vi "Auto 4.vi"(8 "Error In":errorcluster) -> (0 "Error Out":errorcluster)   [LabVIEW 2014]
uses:
  Robot Global Data.vi
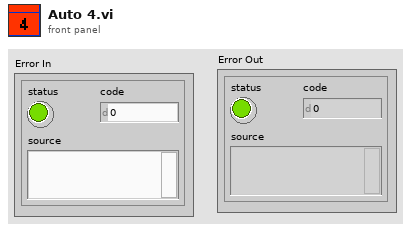
[diagram p1: front panel]
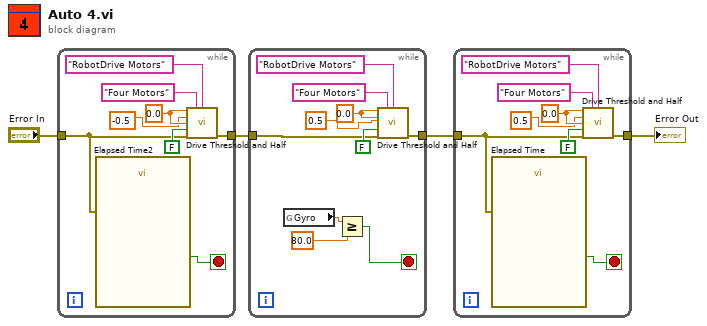
[diagram p0: block diagram]
diagram:
  n1 = while {
    tunnel: "Error In" -> [w5]
    tunnel: [w9] -> w3
    stop <- w6 stop-if-true
    w8 = 0.0 ("Arm Value")
    n2 = call "Elapsed Time2"("error in (no error)"=w5) -> ("Time has Elapsed"=w6:bool)  [unwired: 11 in, 7 out]
    n3 = call "Drive Threshold and Half.vi"("X In"=w8, "Drive refnum name"="Four Motors" ("refnum name"), "Send to DB Name"="RobotDrive Motors" ("Name"), "Y In"=-0.5 ("X In"), "R In"=w8, "Speed Toggle"=FALSE ("Grabber Open/Close"), "Error In"=w5) -> ("Error Out"=w9:errorcluster)  [unwired: 8 in]
  }
  n4 = while {
    tunnel: w3 -> [w19]
    tunnel: [w18] -> w4
    stop <- w13 stop-if-true
    w17 = 0.0 ("Arm Value")
    n5 = global read "Robot Global Data.vi" "Gyro"() -> (w15:dbl)
    n6 = Greater Or Equal?(x=w15, y=80.0) -> (x >= y?=w13:bool)
    n7 = call "Drive Threshold and Half.vi"("X In"=w17, "Drive refnum name"="Four Motors" ("refnum name"), "Send to DB Name"="RobotDrive Motors" ("Name"), "Y In"=w17, "R In"=0.5 ("X In"), "Speed Toggle"=FALSE ("Grabber Open/Close"), "Error In"=w19) -> ("Error Out"=w18:errorcluster)  [unwired: 8 in]
  }
  n8 = while {
    tunnel: w4 -> [w23]
    tunnel: [w27] -> w1
    stop <- w24 stop-if-true
    w26 = 0.0 ("Arm Value")
    n9 = call "Elapsed Time"("error in (no error)"=w23) -> ("Time has Elapsed"=w24:bool)  [unwired: 11 in, 7 out]
    n10 = call "Drive Threshold and Half.vi"("X In"=w26, "Drive refnum name"="Four Motors" ("refnum name"), "Send to DB Name"="RobotDrive Motors" ("Name"), "Y In"=0.5 ("X In"), "R In"=w26, "Speed Toggle"=FALSE ("Grabber Open/Close"), "Error In"=w23) -> ("Error Out"=w27:errorcluster)  [unwired: 8 in]
  }
  "Error Out" <- w1
